vi "Producer.vi"() -> (3 "channel":T1)   [LabVIEW 2023]
doc: "A subVI that produces a triangle wave of 100 values and outputs those values over a channel wire for consumption by a parallel consumer."
uses:
  <extravilib>/ChannelInstances/Stream-i32/)Channel.ctl
  <extravilib>/ChannelInstances/Stream-i32/Write With Abort.vi
  <extravilib>/ChannelInstances/Stream-i32/Endpoint.vi
  <extravilib>/ChannelInstances/Stream-i32/)Channel.vi
  <resource>/ChannelSupport/_ChannelSupport/WaitIfNeeded.vi
  <extravilib>/ChannelInstances/Stream-i32.lvlib
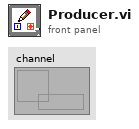
[diagram p1: front panel]
types:
  T1 = typedef "Stream-i32.lvlib/)Channel.ctl" = refnum<queue>
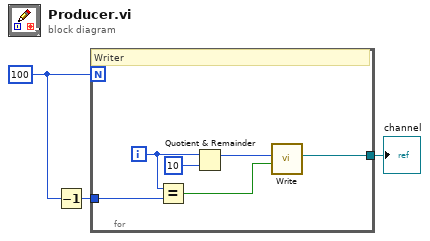
[diagram p0: block diagram]
diagram:
  w2 = 100
  n1 = Decrement(x=w2) -> (x-1=w3:i32)
  n2 = for {
    N: w2 -> [_]
    tunnel: [w4] -> w1
    tunnel: w3 -> [w7]
    i -> [w8]
    # "Writer"
    n3 = Equal?(x=w8, y=w7) -> (x = y?=w5:bool)
    n4 = Quotient & Remainder(x=w8, y=10) -> (x-y*floor(x/y)=w6:i32)  [unwired: 1 out]
    n5 = call <extravilib>:"Write.vi"("last element? (F)"=w5, "element"=w6) -> ("channel"=w4:T1)  [unwired: 7 in, 2 out]
  }
  "channel" <- w1
